vi "Configure Current Peak Low Limit.vi"(0 "VISA resource name":refnum<visa-resource-name>, 5 "Current Peak Low Limit (0 A)":dbl min=0.0 max=152.0 format="%.1f", 11 "Error In":errorcluster) -> (4 "VISA resource name out":refnum<visa-resource-name>, 15 "error out":errorcluster)   [LabVIEW 2014, in "eec 6700.lvlib"]
doc: "Sets the <B>Current Peak Low Limit</B> in the active step of the power source instrument.\n\n<B>Range</B> : 0.000~134.4 A\n\n0.0 ~16.8 A - 6705\n0.0 ~33.6 A - 6710\n0.0 ~67.2 A - 6720\n0.0 ~100.8 A - 6730\n0.0 ~134.4 A - 6740\n\nThe current peak low limit setting configures a minimum peak current threshold or floor level. If a minimum peak current level is not reached a test failure will occur. This insures a load is attached to the power source and there is a minimum peak current present."
uses:
  <instrlib>/eec 6700/eec 6700.lvlib
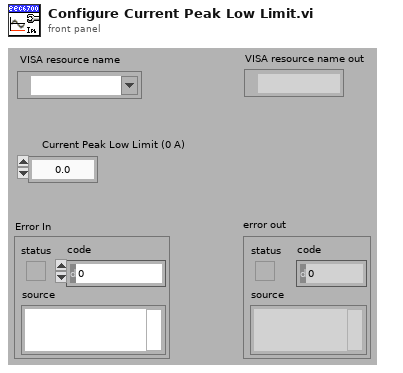
[diagram p1: front panel]
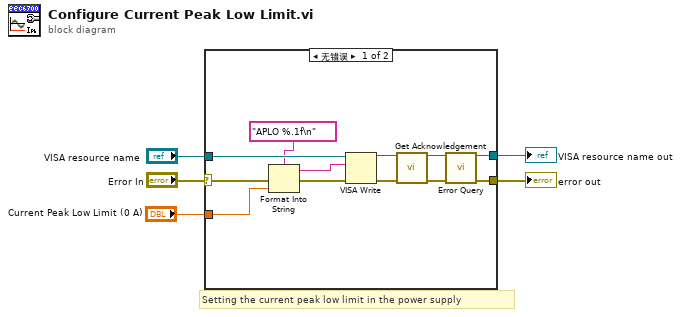
[diagram p0: block diagram]
diagram:
  # "Setting the current peak low limit in the power supply"
  n1 = case shown="无错误" "Error In" {
    selector: "Error In" -> [w11 w19]
    tunnel: "VISA resource name" -> [w17 w18]
    tunnel: [w13 w18] -> w4
    tunnel: [w12 w19] -> w3
    tunnel: "Current Peak Low Limit (0 A)" -> [w16 _]
    frame No Error {
      n2 = Format Into String(format string="APLO %.1f\n" ("Command"), error in=w11, w16) -> (resulting string=w15:string, error out=w10:errorcluster)  [unwired: 1 in]
      n3 = VISA Write(VISA resource name=w17, write buffer=w15, error in (no error)=w10) -> (VISA resource name out=w7:refnum<visa-resource-name>, error out=w6:errorcluster)  [unwired: 1 out]
      n4 = call <instrlib>:"Get Acknowledgement.vi"("VISA resource name"=w7, "error in (no error)"=w6) -> ("VISA resource name out"=w8:refnum<visa-resource-name>, "error out"=w9:errorcluster)  [unwired: 12 in]
      n5 = call <instrlib>:"Error Query.vi"("VISA resource name"=w8, "error in (no error)"=w9) -> ("VISA resource name out"=w13:refnum<visa-resource-name>, "error out"=w12:errorcluster)  [unwired: 10 in, 2 out]
    }
    frame Error {
    }
  }
  "error out" <- w3
  "VISA resource name out" <- w4
